vi "GetScore.vi"(1 "Board in":refnum<class "Board.lvclass">) -> (2 "Score":u32)   [LabVIEW 2021, in "Board.lvclass"]
uses:
  Board.lvclass
  Board.lvclass/Board.ctl
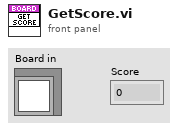
[diagram p1: front panel]
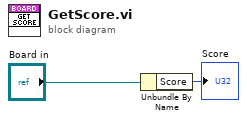
[diagram p0: block diagram]
diagram:
  n1 = Unbundle By Name("Board in") -> ("Score"=→"Score":u32)
